vi "Do.vi"(8 "error in (no error)":errorcluster, 10 "Actor in":refnum<class "Actor.lvclass">, 11 "Auto Probe Sense Value [PAS] Msg":refnum<class "Auto Probe Sense Value [PAS] Msg.lvclass">) -> (0 "error out":errorcluster, 2 "Actor out":refnum<class "Actor.lvclass">)   [LabVIEW 2015, in "CS++Scope.lvlib" / "Auto Probe Sense Value [PAS] Msg.lvclass"]
doc: "This VI delivers the message to the actor by calling the appropriate method(s) on the actor."
uses:
  Auto Probe Sense Value [PAS] Msg.lvclass
  CS++Scope/CS++Scope.lvclass
  <vilib>/ActorFramework/Actor/Actor.lvclass
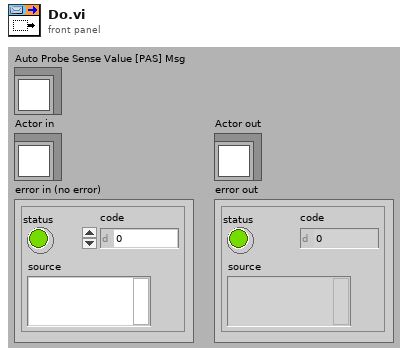
[diagram p1: front panel]
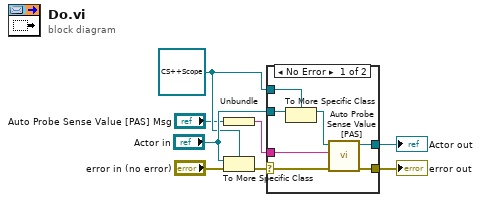
[diagram p0: block diagram]
diagram:
  w3 = refnum<class "CS++Scope.lvclass"> refnum ("Actor in")
  n1 = Unbundle ("Main-Unbundle")("Auto Probe Sense Value [PAS] Msg") -> (w1:string)
  n2 = To More Specific Class(target class=w3, reference="Actor in", error in="error in (no error)") -> (error out=w7:errorcluster)  [unwired: 1 out]
  n3 = case shown="No Error" w7 {
    selector: w7 -> [w13 w17]
    tunnel: [w15 w17] -> w6
    tunnel: [w14 w16] -> w5
    tunnel: "Actor in" -> [w12 w16]
    tunnel: w3 -> [w11 _]
    tunnel: w1 -> [w9 _]
    frame No Error {
      n4 = To More Specific Class(target class=w11, reference=w12) -> (specific class reference=w10:refnum<class "CS++Scope.lvclass">)  [unwired: 1 in, 1 out]
      n5 = call "Auto Probe Sense Value [PAS].vi"("error in (no error)"=w13, "channel name (\"CHANNEL1\")"=w9, "CS++Scope"=w10) -> ("error out"=w15:errorcluster, "CS++Scope out"=w14:refnum<class "CS++Scope.lvclass">)  [unwired: 6 in, 1 out]
    }
    frame Error {
    }
  }
  "error out" <- w6
  "Actor out" <- w5
